vi "sendImageOverNetwork.vi"(8 "error in (no error)":errorcluster, 10 "Image":T1, 11 "Camera in":refnum<class "Camera.lvclass">) -> (0 "error out":errorcluster, 2 "Image out":T1, 3 "Camera out":refnum<class "Camera.lvclass">)   [LabVIEW 2009]
uses:
  Camera.lvclass
  <vilib>/vision/Image Controls.llb/IMAQ Image.ctl
  Tools/Tools.lvlib
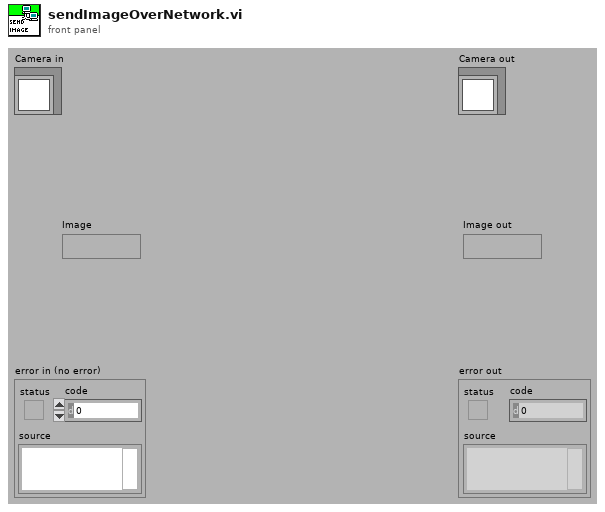
[diagram p1: front panel]
types:
  T1 = typedef "IMAQ Image.ctl" = refnum<image>
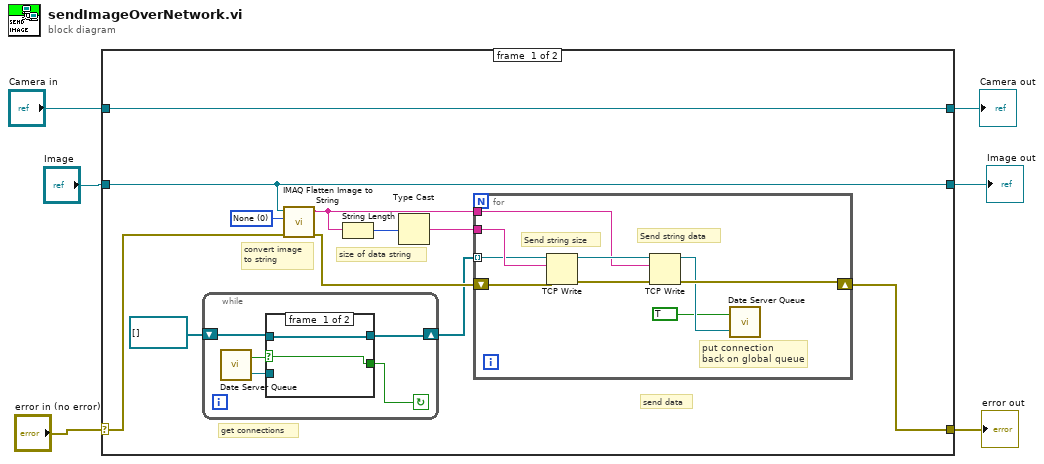
[diagram p0: block diagram]
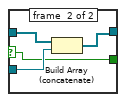
[diagram p2: hidden frame]
diagram:
  n1 = case shown="No Error" "error in (no error)" {
    selector: "error in (no error)" -> [w8 w40]
    tunnel: [w7 w40] -> w5
    tunnel: [w17 w39] -> w3
    tunnel: "Camera in" -> [w17 w39]
    tunnel: "Image" -> [w11 w38]
    tunnel: [w11 w38] -> w1
    frame #0 {
      w12 = 0 items=["None", "JPEG", "PACKED BINARY"]
      # "size of data string"
      # "convert image\nto string"
      # "send data"
      # "get connections"
      n2 = while {
        shift-right: [w27] -> w9
        shift-left: refnum<k5>[] [] ("empty") -> [w28]
        stop <- w29 continue-if-true
        n3 = call "Date Server Queue.vi"() -> ("value"=w30:refnum<k5>, "valid?"=w31:bool)  [unwired: 2 in]
        n4 = case shown="True" w31 {
          selector: w31 -> [w32 w35]
          tunnel: w30 -> [_ w37]
          tunnel: w28 -> [w33 w36]
          tunnel: [w32 w35] -> w29
          tunnel: [w33 w34] -> w27
          frame #0 {
          }
          frame #1 {
            n5 = Build Array (concatenate)(w36, w37) -> (w34:refnum<k5>[])
          }
        }
      }
      n6 = call "IMAQ Flatten Image to String"("error in (no error)"=w8, "Compression (None)"=w12, "Image"=w11) -> ("error out"=w13:errorcluster, "Data String"=w14:string)  [unwired: 7 in]
      n7 = String Length(string=w14) -> (length=w15:i32)
      n8 = Type Cast(x=w15) -> (*(type *) &x=w16:string)  [unwired: 1 in]
      n9 = for {
        tunnel: w16 -> [w24]
        tunnel: w14 -> [w23]
        tunnel: w9 -> [w21] mode=indexing
        shift-right: [w20] -> w7
        shift-left: w13 -> [w22]
        # "put connection\nback on global queue"
        # "Send string data"
        # "Send string size"
        n10 = TCP Write(connection ID=w21, data in=w24, error in (no error)=w22) -> (connection ID out=w25:refnum<k5>, error out=w26:errorcluster)  [unwired: 1 in, 1 out]
        n11 = TCP Write(connection ID=w25, data in=w23, error in (no error)=w26) -> (connection ID out=w19:refnum<k5>, error out=w20:errorcluster)  [unwired: 1 in, 1 out]
        n12 = call "Date Server Queue.vi"("new value"=w19, "set queue? (F: de-queue)"=TRUE) -> ()  [unwired: 2 out]
      }
    }
    frame #1 {
    }
  }
  "error out" <- w5
  "Camera out" <- w3
  "Image out" <- w1
